vi "均值.vi"(1 "输入数组":dbl[](array[numeric])) -> (0 "均值":dbl)   [LabVIEW 2017]
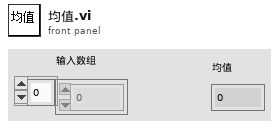
[diagram p1: front panel]
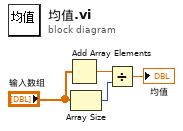
[diagram p0: block diagram]
diagram:
  n1 = Add Array Elements(numeric array="输入数组") -> (sum=w4:dbl)
  n2 = Array Size(array="输入数组") -> (size(s)=w3:i32)
  n3 = Divide(x=w4, y=w3) -> (x/y=→"均值":dbl)
